vi "SLSC_Check Connection and Module.vi"(6 "Connect timeout (s)":dbl=4.0 format="%#_13g", 8 "error in (no error)":errorcluster, 10 "Supported Modules":T1[](array[typedef]), 11 "devices":refnum<k21>) -> (0 "error out":errorcluster, 3 "Device Found?":bool)   [LabVIEW 2019, in "SLSC CD Engine.lvlib"]
uses:
  SLSC CD Engine.lvlib
  SLSC Identification.ctl
  <vilib>/SLSC/Initialize Session with Devices.vi
  <vilib>/SLSC/Close Session.vi
  <vilib>/SLSC/SLSC.lvlib
  <resource>/objmgr/slsc.rc
  SLSC CD Shared/SLSC CD Shared.lvlib
panel:
  out "Supported Modules":T2(array[cluster]) {"Dev.ProductNumber" format="%.0x"; "Dev.VendorNumber" format="%.0x"}
  out "Dev.VendorNum":u32 format="%.0x"
  out "Dev.ProductNum":u32 format="%.0x"
  out "Dev.ProductName":string
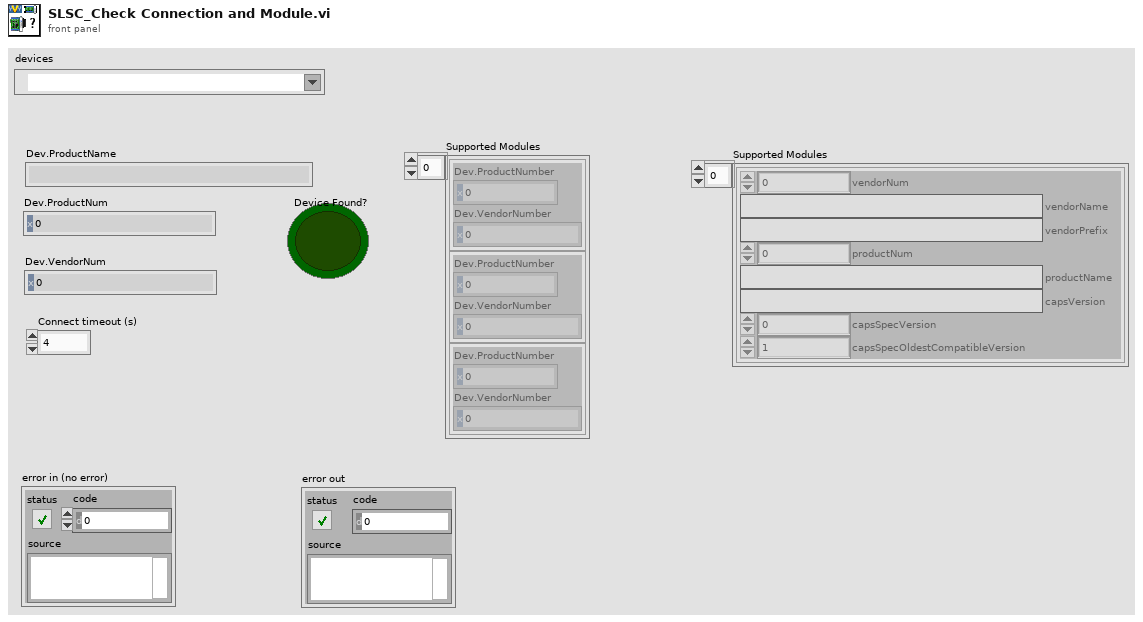
[diagram p1: front panel]
types:
  T1 = typedef "SLSC CD Shared.lvlib/SLSC Identification.ctl" = cluster{"vendorName":string, "productNum":u32, "capsVersion":string, "capsSpecVersion":u32, "productName":string, "vendorNum":u32, "vendorPrefix":string, "capsSpecOldestCompatibleVersion":u32}
  T2 = cluster{"Dev.ProductNumber":u32, "Dev.VendorNumber":u32}[]
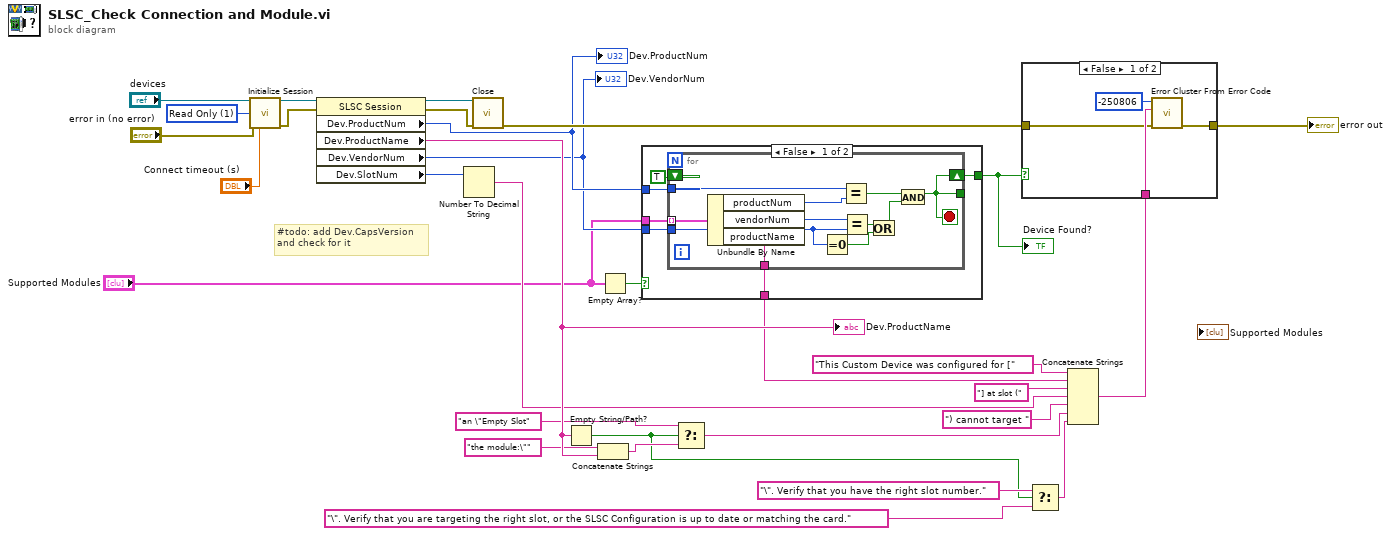
[diagram p0: block diagram]
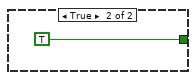
[diagram p2: hidden frame]
diagram:
  w9 = 1 items=["None"=0, "Read Only"=1, "Read/Write"=3] ("reservation access (Read/Write)")
  # "#todo: add Dev.CapsVersion\nand check for it"
  n1 = call-poly <vilib>:"Initialize Session.vi"("devices"="devices", "reservation access (Read/Write)"=w9, "error in (no error)"="error in (no error)", "connect timeout (60 sec)"="Connect timeout (s)") -> ("session out"=w14:refnum<k21>, "error out"=w13:errorcluster)  [unwired: 10 in]
  n2 = property class="SLSC Session"(reference=w14, error in=w13) -> (reference out=w12:refnum<k21>, error out=w11:errorcluster, "Dev.ProductNum"=w19:u32, "Dev.ProductName"=w28:string, "Dev.VendorNum"=w18:u32, "Dev.SlotNum"=w8:u32)
  "Dev.ProductName" <- w28
  "Dev.ProductNum" <- w19
  "Dev.VendorNum" <- w18
  n3 = Number To Decimal String(number=w8) -> (decimal integer string=w15:string)  [unwired: 1 in]
  n4 = call-poly <vilib>:"Close.vi"("session in"=w12, "error in (no error)"=w11) -> ("error out"=w31:errorcluster)  [unwired: 13 in]
  n5 = Empty String/Path?(string/path=w28) -> (empty?=w20:bool)
  n6 = Concatenate Strings("the module:\"" ("error message (\"\")"), w28) -> (w26:string)
  n7 = Empty Array?(array="Supported Modules") -> (empty?=w10:bool)
  n8 = case shown="False" w10 {
    tunnel: w19 -> [w36 _]
    tunnel: "Supported Modules" -> [w35 _]
    tunnel: w18 -> [w34 _]
    tunnel: [w33 TRUE] -> w2
    tunnel: [w32 _] -> w3
    frame False {
      n9 = for {
        tunnel: w36 -> [w48]
        tunnel: w35 -> [w39] mode=indexing
        tunnel: [w44] -> _
        shift-right: [w44] -> w33
        shift-left: TRUE ("x = y?") -> [_]
        tunnel: w34 -> [w43]
        tunnel: [w38] -> w32
        stop <- w44 stop-if-true
        n10 = Unbundle By Name(w39) -> ("productNum"=w46:u32, "vendorNum"=w45:u32, "productName"=w38:string)
        n11 = Equal To 0?(x=w43) -> (x = 0?=w41:bool)
        n12 = Equal?(x=w48, y=w46) -> (x = y?=w47:bool)
        n13 = Equal?(x=w45, y=w43) -> (x = y?=w42:bool)
        n14 = Or(x=w42, y=w41) -> (x .or. y?=w40:bool)
        n15 = And(x=w47, y=w40) -> (x .and. y?=w44:bool)
      }
    }
    frame True {
    }
  }
  "Device Found?" <- w2
  n16 = Select(t="an \"Empty Slot" ("error message (\"\")"), s=w20, f=w26) -> (s? t:f=w27:string)
  n17 = Select(t="\". Verify that you have the right slot number." ("string"), s=w20, f="\". Verify that you are targeting the right slot, or the SLSC Configuration is up to date or matching the card." ("string")) -> (s? t:f=w21:string)
  n18 = Concatenate Strings("This Custom Device was configured for [" ("error message (\"\")"), w3, "] at slot (" ("error message (\"\")"), w15, ") cannot target " ("error message (\"\")"), w27, w21) -> (w30:string)
  n19 = case shown="False" w2 {
    tunnel: [w53 w54] -> w1
    tunnel: w31 -> [w50 w54]
    tunnel: w30 -> [w51 _]
    frame False {
      n20 = call <vilib>:"Error Cluster From Error Code.vi"("error in (no error)"=w50, "error message (\"\")"=w51, "error code (0)"=-250806) -> ("error out"=w53:errorcluster)  [unwired: 6 in]
    }
    frame True {
    }
  }
  "error out" <- w1
